vi "Finalize.vi"(8 "error in (no error)":errorcluster, 11 "Data Plugin in":refnum<class "Data Plugin.lvclass">) -> (0 "error out":errorcluster, 3 "Data Plugin out":refnum<class "Data Plugin.lvclass">)   [LabVIEW 2017, in "Data Engine.lvlib" / "Data Plugin.lvclass"]
uses:
  Data Plugin.lvclass
  Data Plugin.lvclass/Data Plugin.ctl
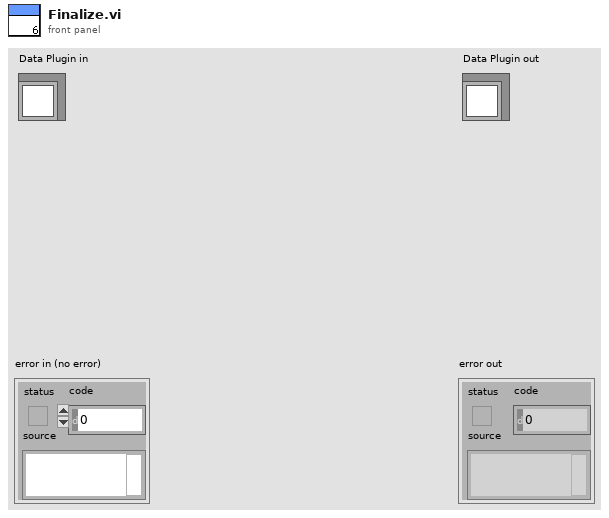
[diagram p1: front panel]
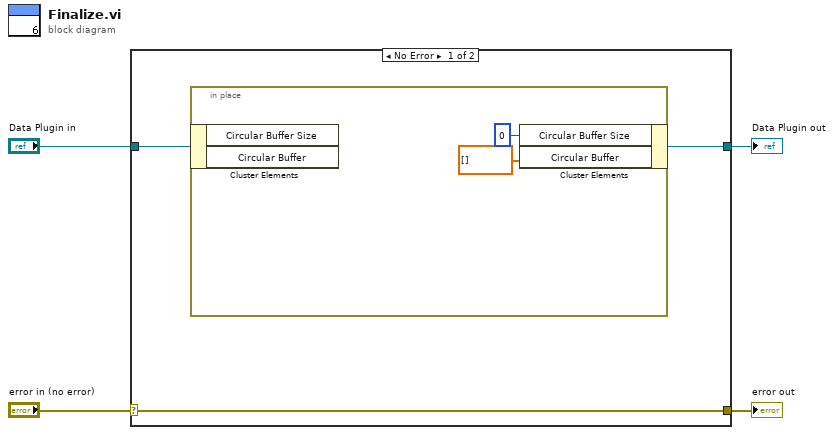
[diagram p0: block diagram]
diagram:
  n1 = case shown="No Error" "error in (no error)" {
    selector: "error in (no error)" -> [w7 w11]
    tunnel: [w7 w11] -> w3
    tunnel: [w5 w10] -> w1
    tunnel: "Data Plugin in" -> [w6 w10]
    frame No Error {
      n2 = in-place {
        n3 = in-place-cluster #1(w6) -> ()  [unwired: 2 out]
        n4 = in-place-cluster #1("Circular Buffer Size"=0, "Circular Buffer"=dbl[] []) -> (w5:refnum<class "Data Plugin.lvclass">)
      }
    }
    frame Error {
    }
  }
  "error out" <- w3
  "Data Plugin out" <- w1
